vi "WhatColorAmIOn.vi"(9 "Metallic Materials Color":string(combo), 10 "Ceramic Materials Color":string(combo), 11 "Organic Materials Color":string(combo)) -> (3 "Drop Off Zone Type":string)   [LabVIEW 2016, in "LEGO-PMR.lvrbt"]
uses:
  LEGO-PMR.lvrbt
  <vilib>/NXT/Block Support/NXT_InputPort.ctl
  <vilib>/NXT/Dual Mode Library/Sensors/EV3_Color_Color.vi
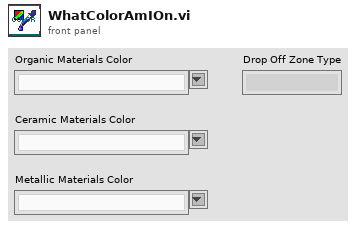
[diagram p1: front panel]
types:
  T1 = typedef "NXT_InputPort.ctl" = u32
  T2 = typedef "ColorSensorColors.ctl" = enum16{"No Color", "Black", "Blue", "Green", "Yellow", "Red", "White", "Brown"}
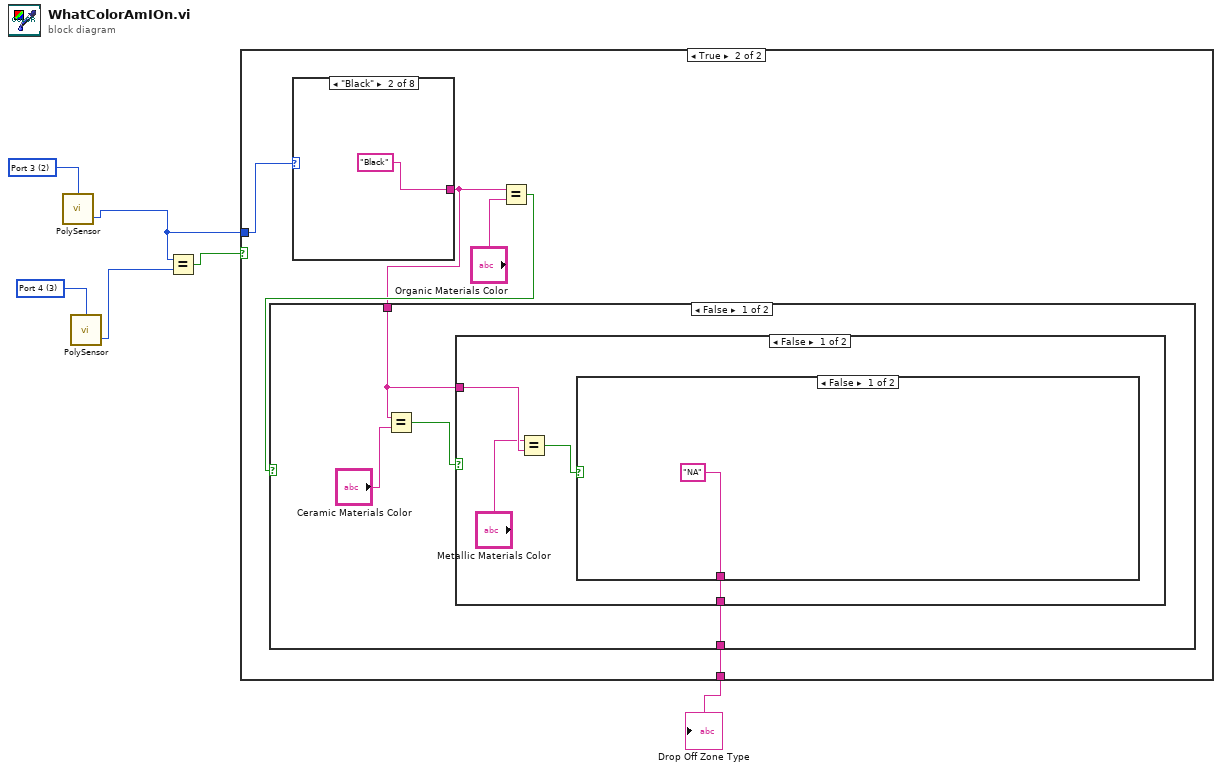
[diagram p0: block diagram]
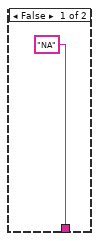
[diagram p2: hidden frame]
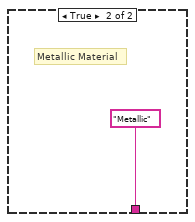
[diagram p3: hidden frame]
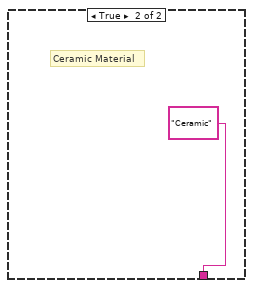
[diagram p4: hidden frame]
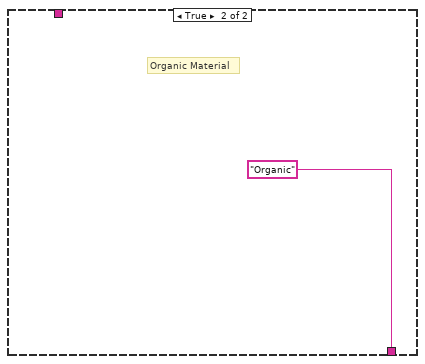
[diagram p5: hidden frame]
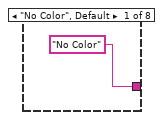
[diagram p6: hidden frame]
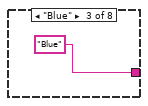
[diagram p7: hidden frame]
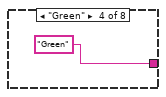
[diagram p8: hidden frame]
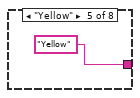
[diagram p9: hidden frame]
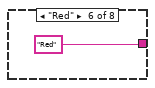
[diagram p10: hidden frame]
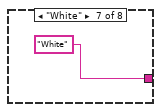
[diagram p11: hidden frame]
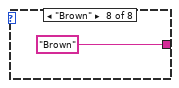
[diagram p12: hidden frame]
diagram:
  w5 = T1 3 items=["Port 1", "Port 2", "Port 3", "Port 4"] ("Port (Port 1)")
  w6 = T1 2 items=["Port 1", "Port 2", "Port 3", "Port 4"] ("Port (Port 1)")
  n1 = call-poly <vilib>:"PolySensor.vi"("Port (Port 1)"=w6) -> ("Detected Color"=w2:T2)  [unwired: 2 in, 1 out]
  n2 = call-poly <vilib>:"PolySensor.vi"("Port (Port 1)"=w5) -> ("Detected Color"=w4:T2)  [unwired: 2 in, 1 out]
  n3 = Equal?(x=w2, y=w4) -> (x = y?=w3:bool)
  n4 = case shown="True" w3 {
    tunnel: w2 -> [_ w12]
    tunnel: ["NA" w8] -> w1
    frame False {
    }
    frame True {
      n5 = case shown="\"Black\"" w12 {
        tunnel: ["No Color" "Black" "Blue" "Green" "Yellow" "Red" "White" "Brown"] -> w9
        frame "No Color", Default {
        }
        frame "Black" {
        }
        frame "Blue" {
        }
        frame "Green" {
        }
        frame "Yellow" {
        }
        frame "Red" {
        }
        frame "White" {
        }
        frame "Brown" {
        }
      }
      n6 = Equal?(x=w9, y="Organic Materials Color") -> (x = y?=w10:bool)
      n7 = case shown="False" w10 {
        tunnel: w9 -> [w14 _]
        tunnel: [w13 "Organic"] -> w8
        frame False {
          n8 = Equal?(x=w14, y="Ceramic Materials Color") -> (x = y?=w15:bool)
          n9 = case shown="False" w15 {
            tunnel: w14 -> [w20 _]
            tunnel: [w17 "Ceramic"] -> w13
            frame False {
              n10 = Equal?(x="Metallic Materials Color", y=w20) -> (x = y?=w18:bool)
              n11 = case shown="False" w18 {
                tunnel: ["NA" "Metallic"] -> w17
                frame False {
                }
                frame True {
                  # "Metallic Material"
                }
              }
            }
            frame True {
              # "Ceramic Material"
            }
          }
        }
        frame True {
          # "Organic Material"
        }
      }
    }
  }
  "Drop Off Zone Type" <- w1
